vi "MoveServos_Ryan.vi"(8 "servo error in":errorcluster, 9 "Y pos":dbl(slide)=136.3265306122449 scale=0.0..180.0, 10 "X pos":dbl(slide)=107.31292517006803 step=0.1 scale=0.0..180.0 scale format="%#.2g", 11 "Device In":i32) -> (0 "servo error out":errorcluster, 3 "Device Out":i32)   [LabVIEW 2014]
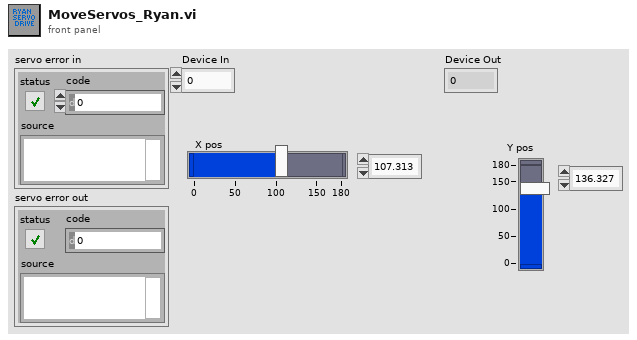
[diagram p1: front panel]
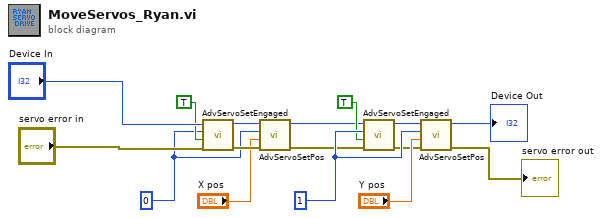
[diagram p0: block diagram]
diagram:
  w7 = 1
  w8 = 0
  n1 = call "AdvServoSetEngaged.vi"("error in (no error)"="servo error in", "SetEngaged"=TRUE, "index"=w8, "Device In"="Device In") -> ("error out"=w10:errorcluster, "Device Out"=w11:i32)  [unwired: 5 in]
  n2 = call "AdvServoSetPos.vi"("error in (no error)"=w10, "pos_in"="X pos", "index"=w8, "Device In"=w11) -> ("error out"=w1:errorcluster, "Device Out"=w2:i32)  [unwired: 5 in]
  n3 = call "AdvServoSetEngaged.vi"("error in (no error)"=w1, "SetEngaged"=TRUE, "index"=w7, "Device In"=w2) -> ("error out"=w5:errorcluster, "Device Out"=w4:i32)  [unwired: 5 in]
  n4 = call "AdvServoSetPos.vi"("error in (no error)"=w5, "pos_in"="Y pos", "index"=w7, "Device In"=w4) -> ("error out"=→"servo error out":errorcluster, "Device Out"=→"Device Out":i32)  [unwired: 5 in]
